vi "10 ms Timer.vi"() -> (2 "10 ms?":bool)   [LabVIEW 2015]
doc: "Outputs a TRUE value every 10 ms."
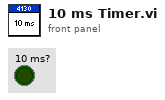
[diagram p1: front panel]
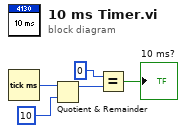
[diagram p0: block diagram]
diagram:
  n1 = Tick Count (ms)() -> (millisecond timer value=w2:u32)
  n2 = Quotient & Remainder(x=w2, y=u32 10) -> (x-y*floor(x/y)=w4:u32)  [unwired: 1 out]
  n3 = Equal?(x=u32 0, y=w4) -> (x = y?=→"10 ms?":bool)
